vi "Chronometer.vi"(11 "Action in":enum16{"Count", "Stop", "Reset"}(ring)) -> (1 "Second":i32, 2 "Fractional Second":dbl format="%#.4g", 3 "Time":dbl, 4 "Minute":i32, 5 "Hour":i32, 6 "Action out":enum16{"Count", "Stop", "Reset"}(ring))   [LabVIEW 2015]
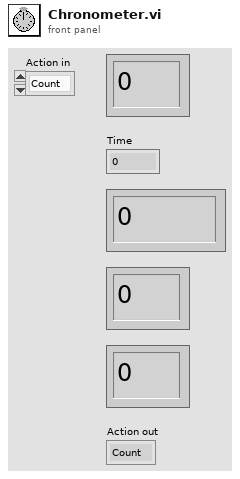
[diagram p1: front panel]
types:
  T1 = cluster{"Start":bool, "Pause":bool, "Reset":bool}
  T2 = typedef "LVDateTimeRec.ctl" = cluster{"fractional second":dbl, "second":i32, "minute":i32, "hour":i32, "day of month":i32, "month":i32, "year":i32, "day of week":i32, "day of year":i32, "DST":i32}
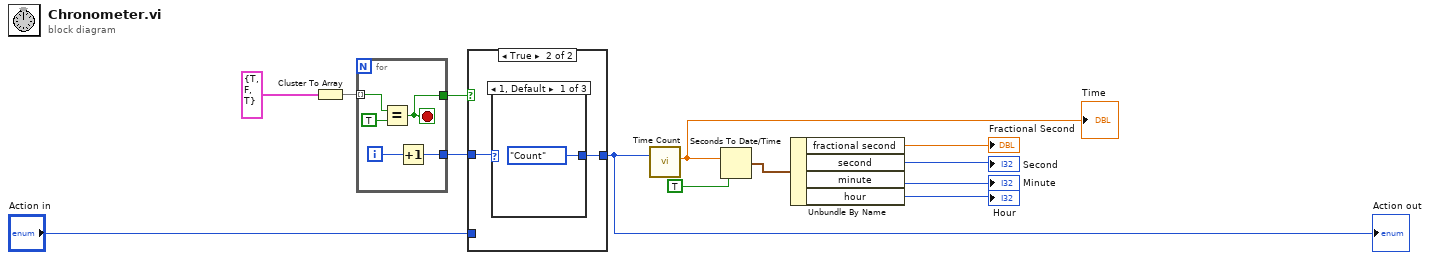
[diagram p0: block diagram]
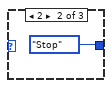
[diagram p3: hidden frame]
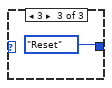
[diagram p4: hidden frame]
diagram:
  n1 = Cluster To Array(cluster=T1 {"Start"=TRUE, "Pause"=FALSE, "Reset"=TRUE} ("Buttons")) -> (array=w3:bool[])
  n2 = for {
    tunnel: w3 -> [w17] mode=indexing
    tunnel: [w15] -> w2
    tunnel: [w14] -> w1
    i -> [w16]
    stop <- w14 stop-if-true
    n3 = Equal?(x=w17, y=TRUE) -> (x = y?=w14:bool)
    n4 = Increment(x=w16) -> (x+1=w15:i32)
  }
  n5 = case shown="True" w1 {
    tunnel: w2 -> [_ w21]
    tunnel: "Action in" -> [w19 _]
    tunnel: [w19 w20] -> w6
    frame False {
    }
    frame True {
      n6 = case shown="1, Default" w21 {
        tunnel: [enum16{"Count", "Stop", "Reset"}."Count" ("Action") enum16{"Count", "Stop", "Reset"}."Stop" ("Action") enum16{"Count", "Stop", "Reset"}."Reset" ("Action")] -> w20
        frame 1, Default {
        }
        frame 2 {
        }
        frame 3 {
        }
      }
    }
  }
  "Action out" <- w6
  n7 = call "Time Count.vi"("Action"=w6) -> ("Time"=w10:dbl)  [unwired: 10 in]
  "Time" <- w10
  n8 = Seconds To Date/Time(time stamp (now)=w10, to UTC (F)=TRUE) -> (date time rec=w8:T2)
  n9 = Unbundle By Name(w8) -> ("fractional second"=→"Fractional Second":dbl, "second"=→"Second":i32, "minute"=→"Minute":i32, "hour"=→"Hour":i32)
